vi "MoveArmForTime-C.vi"(11 "Params":string[][](array[string])) -> ()   [LabVIEW 2017]
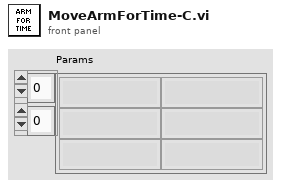
[diagram p1: front panel]
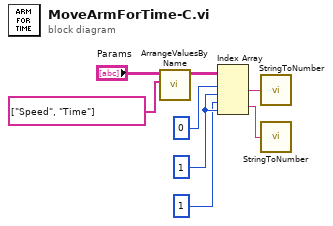
[diagram p0: block diagram]
diagram:
  w6 = 1
  n1 = call "ArrangeValuesByName.vi"("Names"=string[] ["Speed", "Time"], "Names/Values in"="Params") -> ("Names/Values Out"=w7:string[][])  [unwired: 9 in]
  n2 = Index Array(array=w7, index (row) #1=0, index (col) #1=w6, index (row) #2=1, index (col) #2=w6) -> (element #1=w3:string, element #2=w1:string)
  n3 = call "StringToNumber.vi"("String"=w3) -> ()  [unwired: 1 out]
  n4 = call "StringToNumber.vi"("String"=w1) -> ()  [unwired: 1 out]
